vi "SA40289A.20211015 Data Analysis.vi"() -> ()   [LabVIEW 2020]
uses:
  <vilib>/Analysis/baseanly.llb/Mean (DBL).vi
  <userlib>/_OpenG.lib/file/file.llb/Build Path - Traditional__ogtk.vi
  <userlib>/LevyLab/XY Utilities/subVIs/Linear Fit (multiple).vi
  <userlib>/LevyLab/XY Utilities/subVIs/Get X and Y (multiple).vi
  <userlib>/LevyLab/LV to ITX/Data/Data.lvclass
  <userlib>/LevyLab/XY Utilities/xy_utilities.lvlib
  <vilib>/Analysis/NI_AALBase.lvlib
panel:
  out "Environment":enum16{"Air/Helium", "Vacuum"}(ring)
  out "Increasing Temp?":bool
  out "E_a":dbl[](array[numeric])
  in  "Tab Control":enum32{"2T data", "1D, 2D, and 4T Data"}(tab)
  out "G2T vs t":T1(graph)
  out "Temp vs t":T1(graph)
  out "G2T Slopes vs Temp":T1(graph)
  out "Arrhenius":T1(graph)
  out "G4T vs t 2D":T1(graph)
  out "G4T vs t 1D":T1(graph)
  out "Temp vs t 2":T1(graph)
  in  "One File?":bool
  in  "Arrhenius?":bool
  in  "2D Data?":bool=TRUE
  in  "Source Voltage":dbl=0.1
  in  "Init Temp":i32=275
  in  "Temp Step":i32=5
  in  "Final Temp":i32=300
  in  "Data File":path=path "G:/My Drive/ansom/Data (1)/PPMS 2/SA40289.20211015/00 - test/SA40289.20211015.275K.dat"
  in  "Trimming":i32=400
  in  "Update":bool
  in  "OK":bool
  out "error out":errorcluster
  in  "error in (no error)":errorcluster
  # "G2T"
  # "G4T 1D"
  # "G2T"
  # "G4T 2D"
  # "V1-"
  # "I-"
  # "V1+"
  # "V2-"
  # "I+"
  # "V2+"
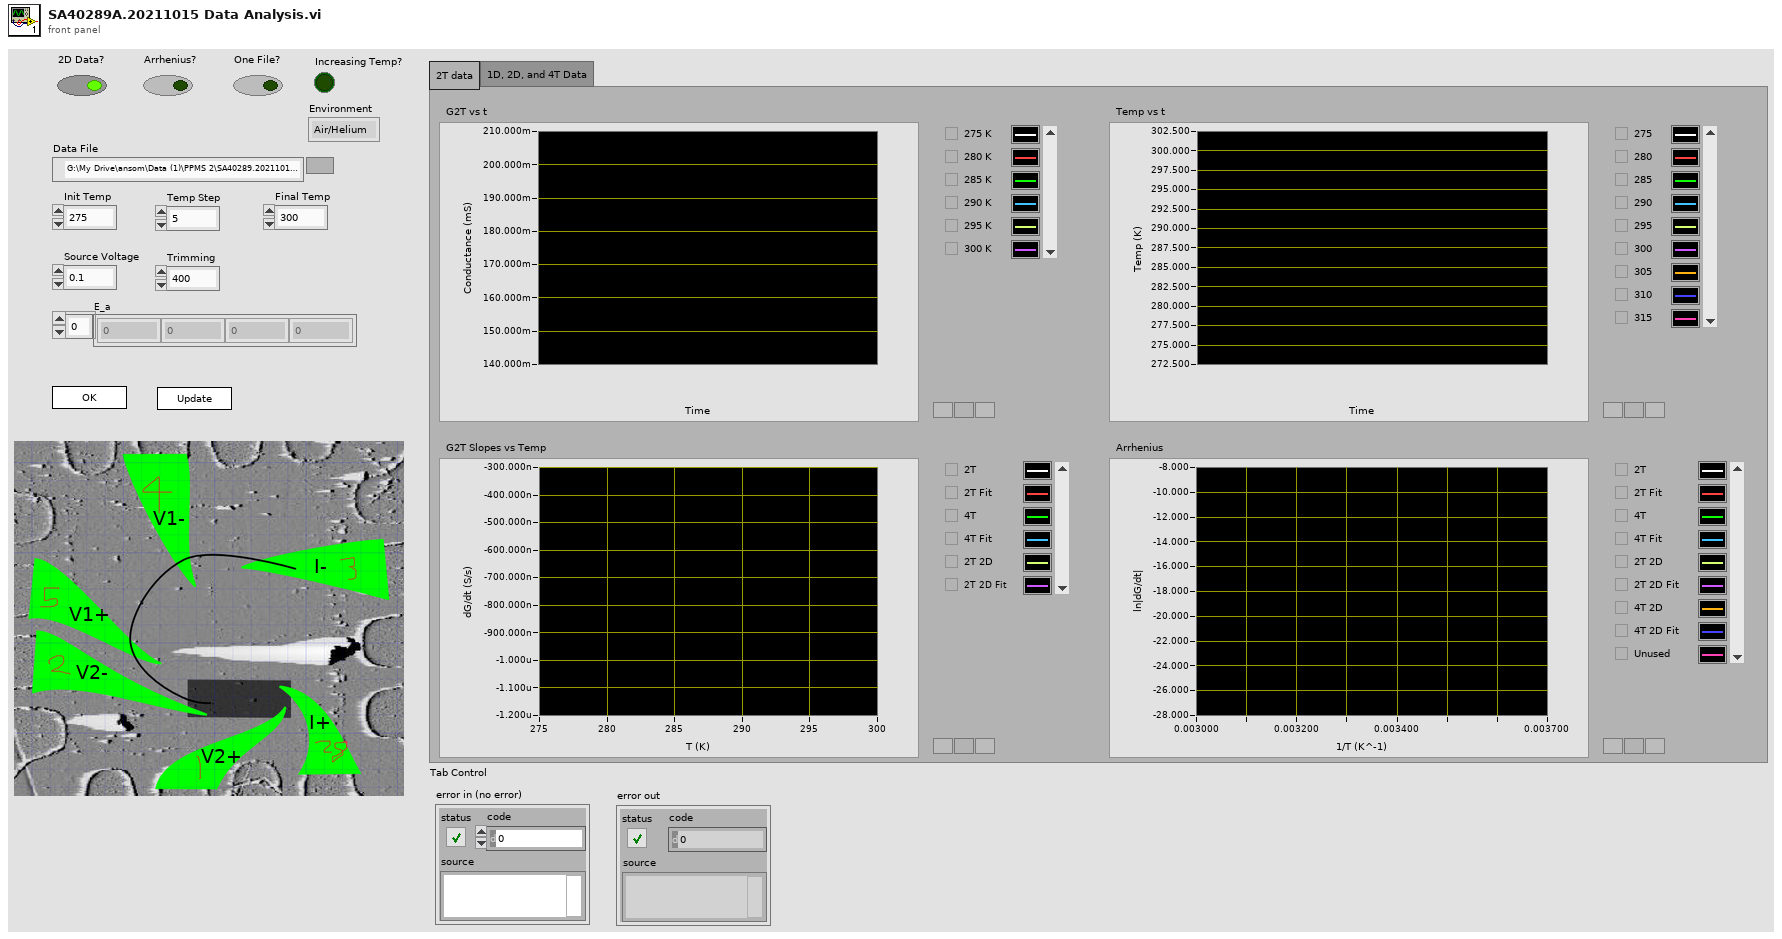
[diagram p1: front panel]
types:
  T1 = cluster{"Data":dbl[], "Best Exponential Fit":dbl[]}[]
  T2 = enum32{"Invalid", "Standard", "Closed", "Hidden", "Minimized", "Maximized"}
  T3 = enum32{"invalid app kind", "Development System", "Run Time System", "Student Edition", "Embedded LabVIEW", "Evaluation", "Custom"}
  T4 = cluster{"Core":cluster{"Current VI Reference":refnum<vi>, "Close Panel on Exit?":bool}, "G2T 1D":cluster{dbl[], dbl[]}[], "G4T 1D":cluster{dbl[], dbl[]}[], "G2T 2D":cluster{dbl[], dbl[]}[], "G4T 2D":cluster{dbl[], dbl[]}[], "Temp":cluster{dbl[], dbl[]}[], "G2T Slopes":cluster{dbl[], dbl[]}[], "Source Voltage":dbl, "Final Temp":i32, "Init Temp":i32, "Temp Step":i32, "Data File":path, "Trimming":i32}
  T5 = cluster{"Current VI Reference":refnum<vi>, "Close Panel on Exit?":bool}
  T6 = typedef "Data.lvclass/Dictionary--cluster.ctl" = cluster{"key":string, "value":variant}
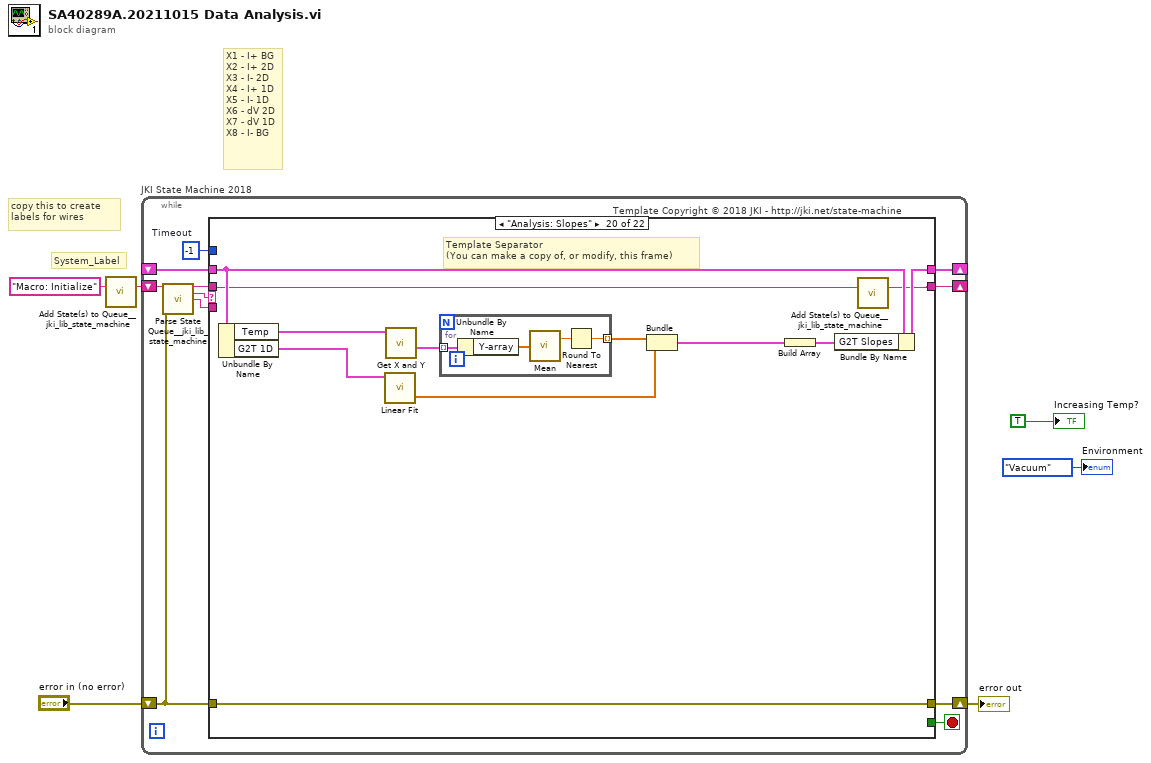
[diagram p0: block diagram]
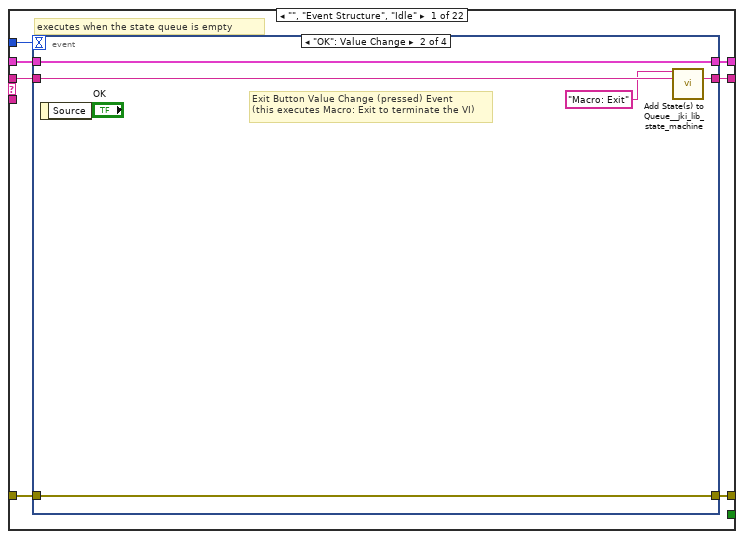
[diagram p2: hidden frame]
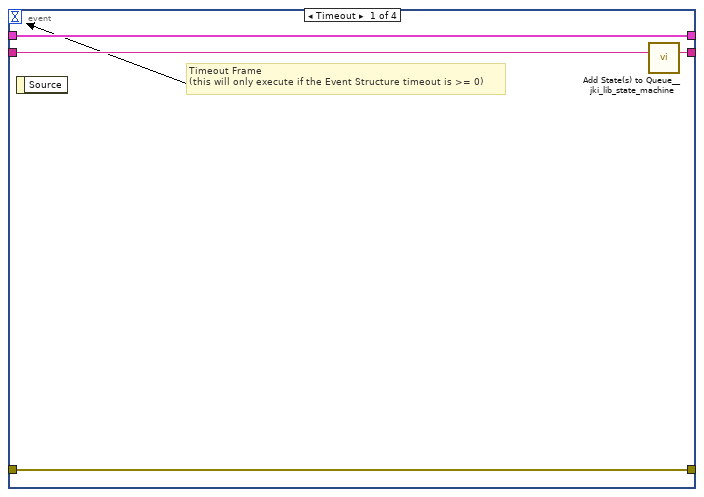
[diagram p3: hidden frame]
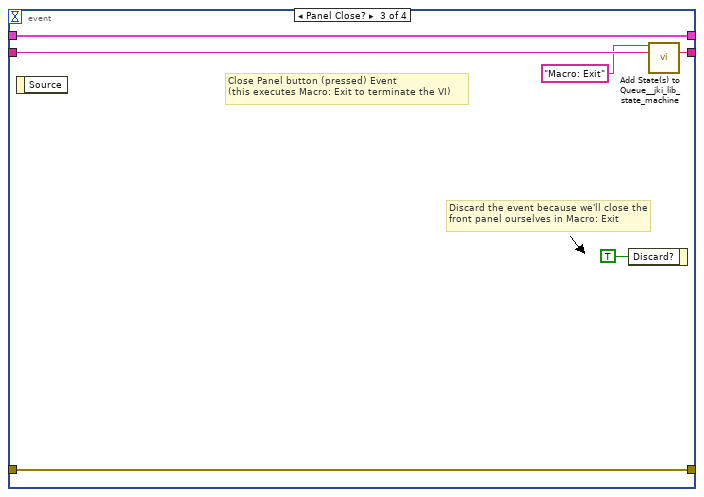
[diagram p4: hidden frame]
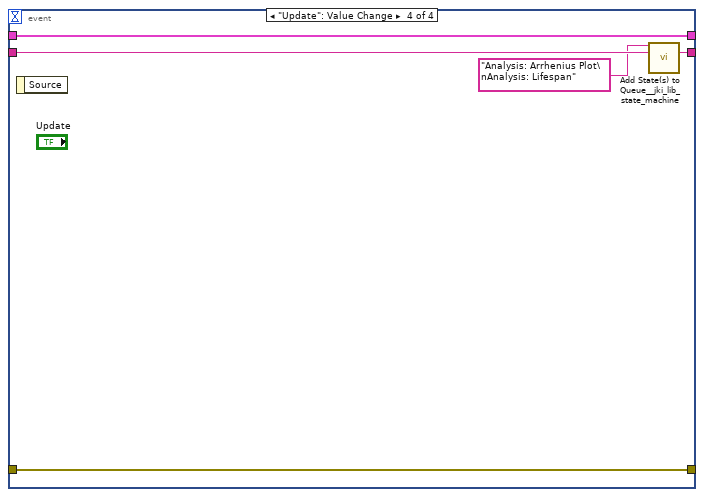
[diagram p5: hidden frame]
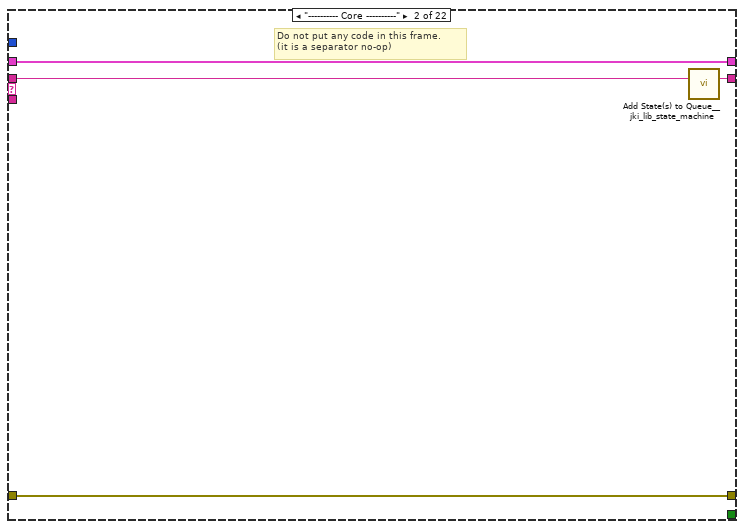
[diagram p6: hidden frame]
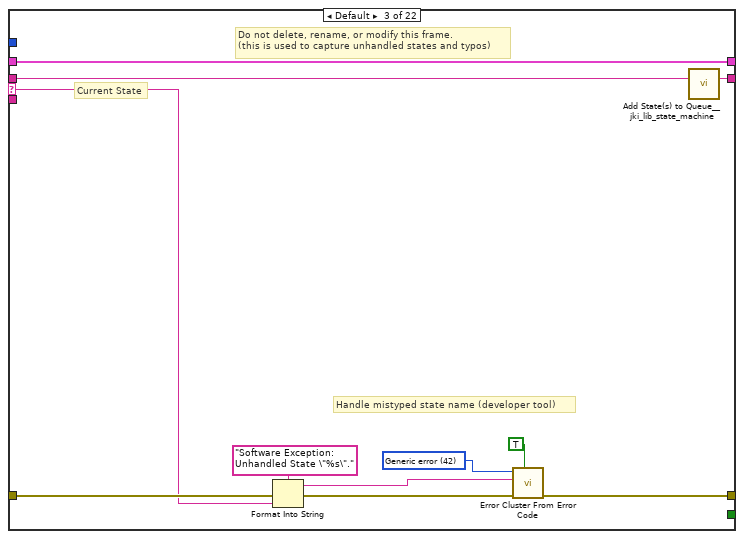
[diagram p7: hidden frame]
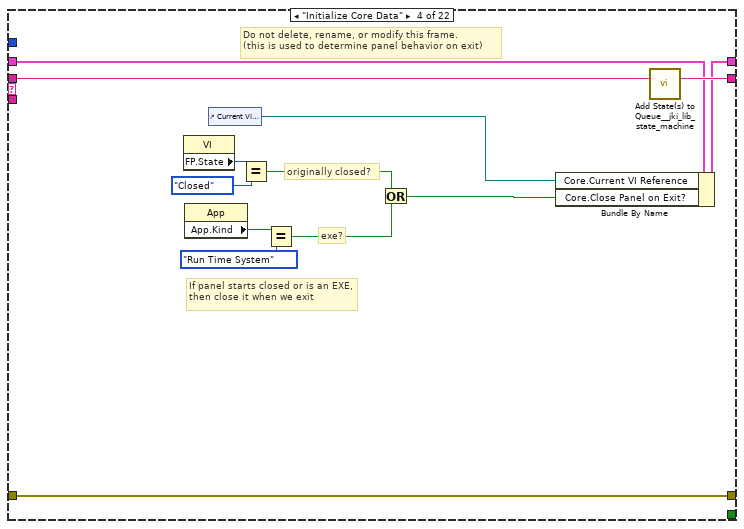
[diagram p8: hidden frame]
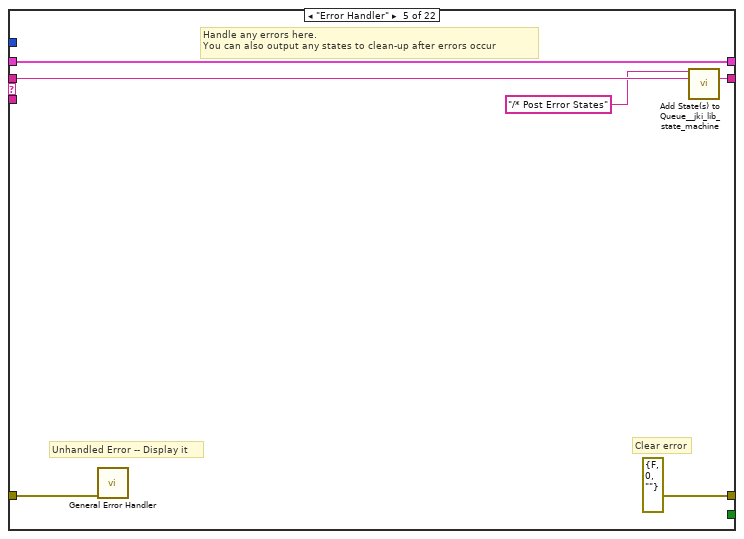
[diagram p9: hidden frame]
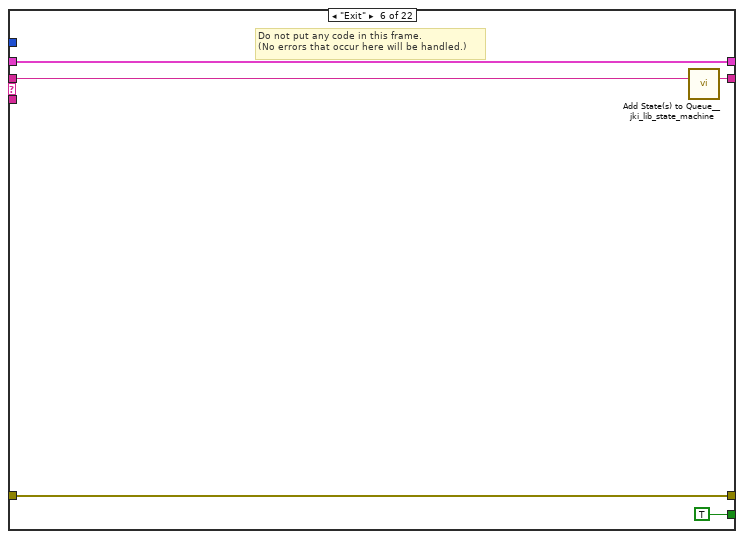
[diagram p10: hidden frame]
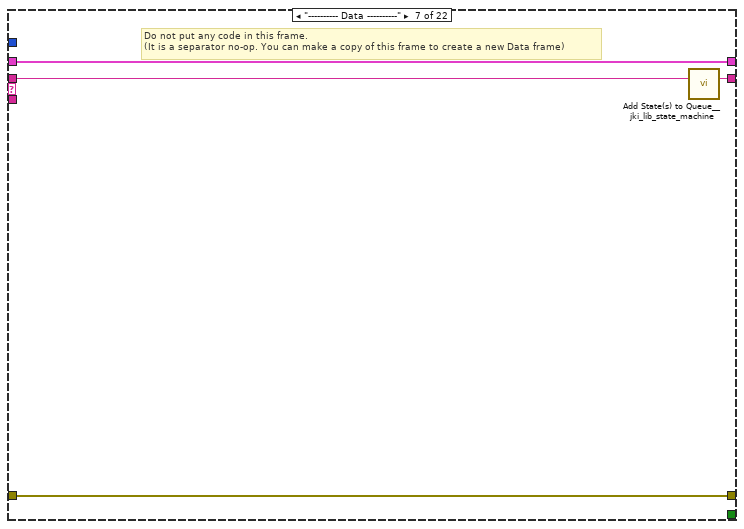
[diagram p11: hidden frame]
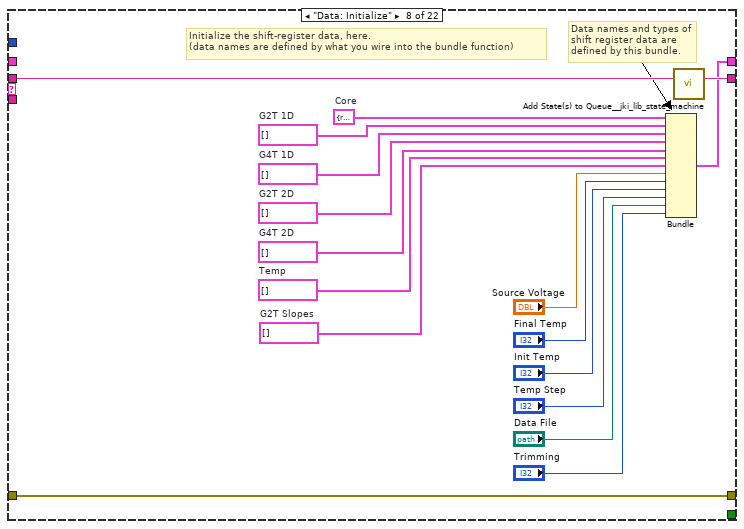
[diagram p12: hidden frame]
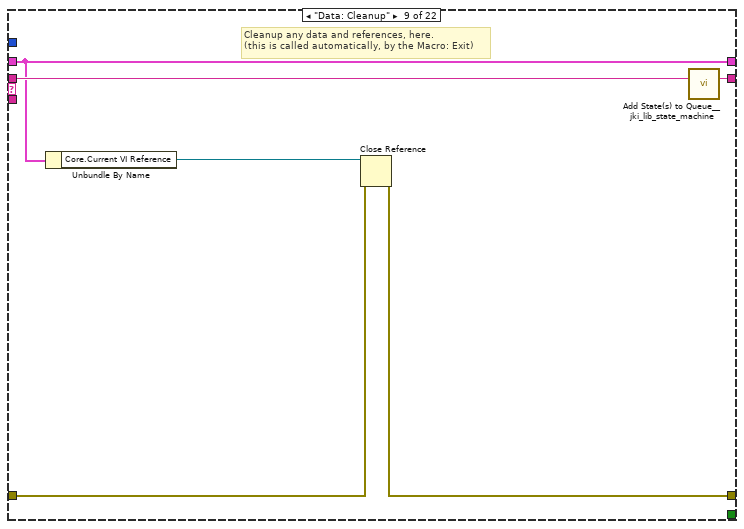
[diagram p13: hidden frame]
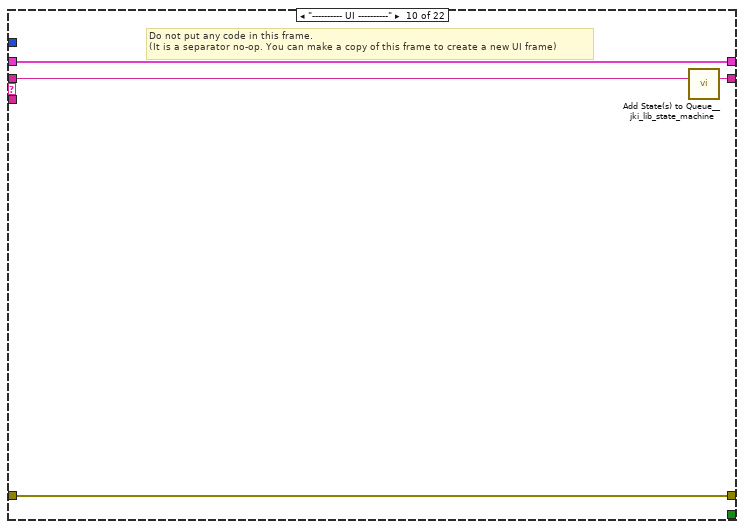
[diagram p14: hidden frame]
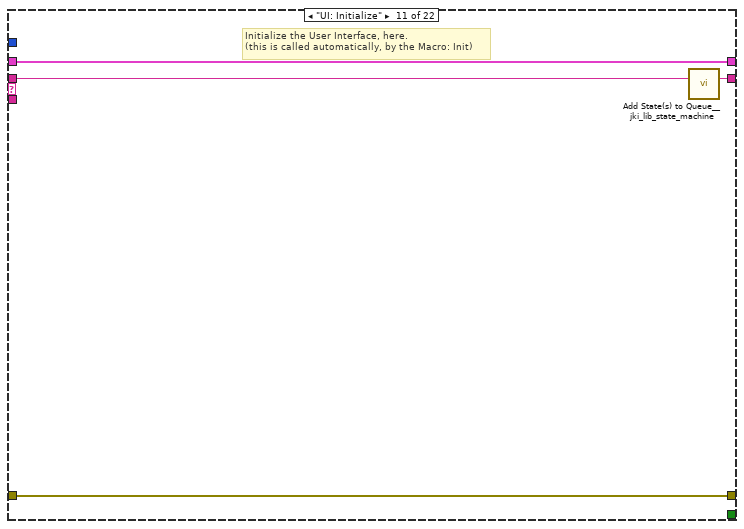
[diagram p15: hidden frame]
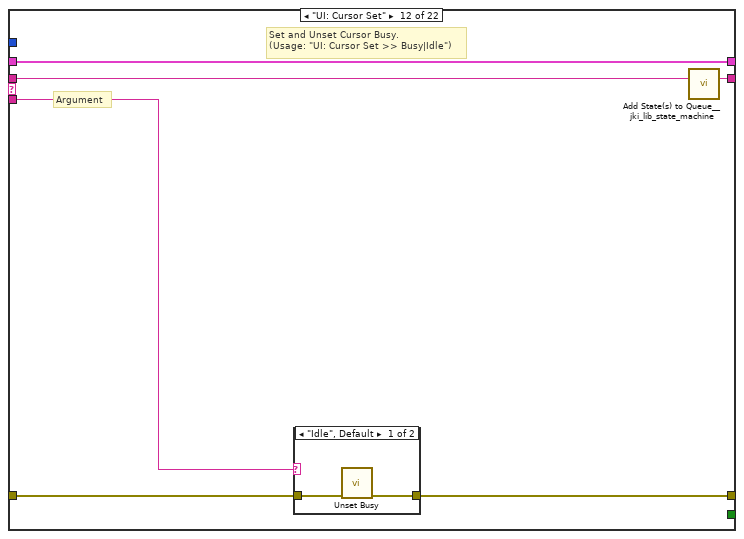
[diagram p16: hidden frame]
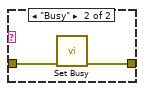
[diagram p17: hidden frame]
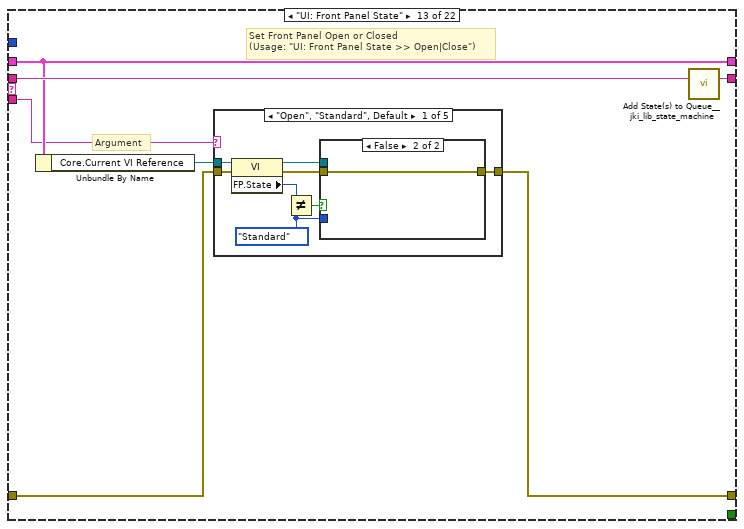
[diagram p18: hidden frame]
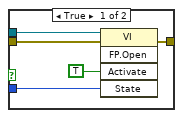
[diagram p19: hidden frame]
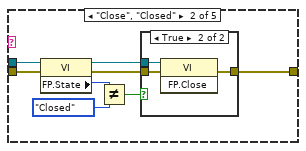
[diagram p20: hidden frame]
diagram:
  # "copy this to create labels for wires"
  # "System_Label"
  # "X1 - I+ BG\nX2 - I+ 2D\nX3 - I- 2D\nX4 - I+ 1D\nX5 - I- 1D\nX6 - dV 2D\nX7 - dV 1D\nX8 - I- BG"
  n1 = call <vilib>:"Add State(s) to Queue__jki_lib_state_machine.vi"("State(s) in (\"\")"="Macro: Initialize") -> ("States Out"=w6:string)  [unwired: 14 in]
  n2 = while "JKI State Machine 2018" {
    shift-right: [w10] -> _
    shift-left: _ -> [w9]
    shift-right: [w13] -> w3
    shift-left: "error in (no error)" -> [w7]
    shift-right: [w12] -> _
    shift-left: w6 -> [w14]
    stop <- w11 stop-if-true
    w8 = -1  # Timeout
    # "Template Copyright © 2018 JKI - http://jki.net/state-machine"
    n3 = call <vilib>:"Parse State Queue__jki_lib_state_machine.vi"("State Queue"=w14, "Error In (no error)"=w7) -> ("Remaining States"=w16:string, "Current State"=w17:string, "Arguments"=w15:string)  [unwired: 11 in]
    n4 = case shown="\"Analysis: Slopes\"" w17 {
      selector: w17 -> [_ _ w49 _ _ _ _ _ _ _ _ _ _ _ _ _ _ _ _ _ _ _]
      tunnel: w16 -> [w24 w48 w53 w72 w78 w83 w87 w104 w110 w114 w118 w124 w135 w204 w219 w229 w233 w250 w322 w371 w388 w446]
      tunnel: w15 -> [_ _ _ _ _ _ _ _ _ _ _ w119 w129 _ _ _ _ _ _ _ _ _]
      tunnel: w9 -> [w22 w45 w51 w65 w75 w81 w84 _ w105 w111 w116 w122 w131 w201 w216 w226 w230 w244 w308 w373 w385 w443]
      tunnel: [w21 w46 w55 w69 errorcluster {"status"=FALSE, "code"=0, "source"=""} ("error out") w80 w85 w101 w106 w112 w115 w120 w132 w202 w217 w227 w231 w246 w320 w375 w386 w444] -> w13
      tunnel: w7 -> [w20 w46 w54 w69 w74 w80 w85 w101 w107 w112 w115 w121 w133 w202 w217 w227 w231 w246 w320 w375 w386 w444]
      tunnel: [w23 w47 w52 w71 w77 w82 w86 w103 w109 w113 w117 w123 w134 w203 w218 w228 w232 w249 w321 w372 w387 w445] -> w12
      tunnel: [_ _ _ _ _ TRUE _ _ _ _ _ _ _ _ _ _ _ _ _ _ _ _] -> w11
      tunnel: [w19 w45 w51 w70 w75 w81 w84 w102 w105 w111 w116 w122 w131 w201 w216 w226 w230 w245 w309 w374 w385 w443] -> w10
      tunnel: w8 -> [w18 _ _ _ _ _ _ _ _ _ _ _ _ _ _ _ _ _ _ _ _ _]
      frame "", "Event Structure", "Idle" {
        # "executes when the state queue is empty"
        n5 = event shown="[1] \"OK\": Value Change" {
          selector: _ -> [_ _ _ _]
          dyn-events: _ -> [_ _ _ _]
          timeout: w18 -> [_ _ _ _]
          tunnel: w24 -> [w28 w33 w39 w43]
          tunnel: [w27 w32 w38 w42] -> w23
          tunnel: w22 -> [w25 w30 w36 w44]
          tunnel: [w26 w31 w37 w40] -> w21
          tunnel: w20 -> [w26 w31 w37 w40]
          tunnel: [w25 w30 w36 w44] -> w19
          event Timeout {
            # "Timeout Frame\n(this will only execute if the Event Structure timeout is >= 0)"
            n6 = event-data() -> ()  [unwired: 1 in, 1 out]
            n7 = call <vilib>:"Add State(s) to Queue__jki_lib_state_machine.vi"("State(s) in (\"\")"=w28) -> ("States Out"=w27:string)  [unwired: 14 in]
          }
          event "OK": Value Change {
            # "Exit Button Value Change (pressed) Event\n(this executes Macro: Exit to terminate the VI)"
            n8 = event-data() -> ()  [unwired: 1 in, 1 out]
            n9 = call <vilib>:"Add State(s) to Queue__jki_lib_state_machine.vi"("State(s) in Front (\"\")"="Macro: Exit", "State(s) in (\"\")"=w33) -> ("States Out"=w32:string)  [unwired: 13 in]
          }
          event Panel Close? {
            # "Discard the event because we'll close the front panel ourselves in Macro: Exit"
            # "Close Panel button (pressed) Event\n(this executes Macro: Exit to terminate the VI)"
            n10 = event-data() -> ()  [unwired: 1 in, 1 out]
            n11 = event-data("Discard?"=TRUE) -> ()  [unwired: 1 in, 1 out]
            n12 = call <vilib>:"Add State(s) to Queue__jki_lib_state_machine.vi"("State(s) in Front (\"\")"="Macro: Exit", "State(s) in (\"\")"=w39) -> ("States Out"=w38:string)  [unwired: 13 in]
          }
          event "Update": Value Change {
            n13 = event-data() -> ()  [unwired: 1 in, 1 out]
            n14 = call <vilib>:"Add State(s) to Queue__jki_lib_state_machine.vi"("State(s) in Front (\"\")"="Analysis: Arrhenius Plot\nAnalysis: Lifespan" ("State(s) in Front (\"\")"), "State(s) in (\"\")"=w43) -> ("States Out"=w42:string)  [unwired: 13 in]
          }
        }
      }
      frame "---------- Core ----------" {
        # "Do not put any code in this frame.\n(it is a separator no-op)"
        n15 = call <vilib>:"Add State(s) to Queue__jki_lib_state_machine.vi"("State(s) in (\"\")"=w48) -> ("States Out"=w47:string)  [unwired: 14 in]
      }
      frame Default {
        w58 = 42 items=["No error", "Argument error", "Memory is full", "Out of zone", "End of file", "File already open", "Generic file I/O error", "File not found", "File permission error", "Disk is full", "Duplicate path", "Too many files open", "System feature not enabled", "Resource file not found", "Cannot add resource", "Resource not found", "Image not found", "Image memory error", "Pen does not exist", "Config type invalid", "Config token not found", "Config parse error", "Config memory error", "Bad external code format", "Bad external code offset", "External code not present", "Null window", "Destroy window error", "Null menu", "Print aborted", "Bad print record", "Print driver error", "Windows error during printing", "Memory error during printing", "Print dialog error", "Generic print error", "Invalid device refnum", "Device not found", "Device parameter error", "Device unit error", "Cannot open device", "Device call aborted", "Generic error", "Cancelled by user", "Object ID too low", "Object ID too high", "Object not in heap", "Unknown heap", "Unknown object (invalid DefProc)", "Unknown object (DefProc not in table)", "Message out of range", "Invalid (null) method", "Unknown message", "Manager call not supported", "Bad address", "Network operation in progress", "Network operation timed out", "Connection is busy", "Network attribute not supported", "Network error", "Address in use", "System out of memory", "Connection aborted", "Connection refused", "Not connected", "Already connected", "Connection closed", "Initialization error (interapplication manager)", "Bad occurrence", "Wait on unbound occurrence handler", "Occurrence queue overflow", "Datalog type conflict", "Unused", "Unrecognized type (interapplication manager)", "Memory corrupt", "Failed to make temporary DLL", "Old CIN version", "Drag socket not found", "Failed to load drop-object", "Failed to register OLE object", "Failed to release OLE object", "Format specifier type mismatch", "Unknown format specifier", "Too few format specifiers", "Too many format specifiers", "Scan failed", "Newer CIN version", "Error converting to variant", "Runtime menu error", "Password tampered", "Variant attribute not found", "Incompatible variant data type", "Event data is not available", "Event Store is not present", "Occurrence is not found", "Event Queue is not created", "Event info is not available", "Refnum passed is NULL", "Error retrieving Class GUID", "Error retrieving CoClass GUID", "Error retrieving TypeLib GUID.", "Bad built application magic bytes.", "Specific driver is different from the specific driver associated with the Logical Name.", "There is no session opened to the class driver.", "Max Error", "MAX - Error with config objects", "MAX - Error loading configuration", "MAX - Group not supported"]
        # "Current State"
        # "Do not delete, rename, or modify this frame.\n(this is used to capture unhandled states and typos)"
        # "Handle mistyped state name (developer tool)"
        n16 = Format Into String(format string="Software Exception: Unhandled State \"%s\"." ("message"), error in=w54, w49) -> (resulting string=w57:string, error out=w56:errorcluster)  [unwired: 1 in]
        n17 = call <vilib>:"Error Cluster From Error Code.vi"("show call chain? (False)"=TRUE, "error in (no error)"=w56, "error message (\"\")"=w57, "error code (0)"=w58) -> ("error out"=w55:errorcluster)  [unwired: 5 in]
        n18 = call <vilib>:"Add State(s) to Queue__jki_lib_state_machine.vi"("State(s) in (\"\")"=w53) -> ("States Out"=w52:string)  [unwired: 14 in]
      }
      frame "Initialize Core Data" {
        # "Do not delete, rename, or modify this frame.\n(this is used to determine panel behavior on exit)"
        # "originally closed?"
        # "exe?"
        # "If panel starts closed or is an EXE, then close it when we exit"
        n19 = property class="VI"() -> ("FP.State"=w62:T2)  [unwired: 2 in, 2 out]
        n20 = property class="App"() -> ("App.Kind"=w68:T3)  [unwired: 2 in, 2 out]
        n21 = control-ref of="Current VI Reference"() -> (w63:refnum<vi>)
        n22 = Equal?(x=w62, y=T2."Closed" ("Front Panel Window:State")) -> (x = y?=w60:bool)
        n23 = Equal?(x=w68, y=T3."Run Time System" ("Application:Kind")) -> (x = y?=w66:bool)
        n24 = Or(x=w60, y=w66) -> (x .or. y?=w64:bool)
        n25 = Bundle By Name(cluster=w65, "Core.Current VI Reference"=w63, "Core.Close Panel on Exit?"=w64) -> (w70:T4)
        n26 = call <vilib>:"Add State(s) to Queue__jki_lib_state_machine.vi"("State(s) in (\"\")"=w72) -> ("States Out"=w71:string)  [unwired: 14 in]
      }
      frame "Error Handler" {
        # "Unhandled Error -- Display it"
        # "Handle any errors here.\nYou can also output any states to clean-up after errors occur"
        # "Clear error"
        n27 = call <vilib>:"General Error Handler.vi"("error in (no error)"=w74) -> ()  [unwired: 10 in, 5 out]
        n28 = call <vilib>:"Add State(s) to Queue__jki_lib_state_machine.vi"("State(s) in Front (\"\")"="/* Post Error States", "State(s) in (\"\")"=w78) -> ("States Out"=w77:string)  [unwired: 13 in]
      }
      frame "Exit" {
        # "Do not put any code in this frame.\n(No errors that occur here will be handled.)"
        n29 = call <vilib>:"Add State(s) to Queue__jki_lib_state_machine.vi"("State(s) in (\"\")"=w83) -> ("States Out"=w82:string)  [unwired: 14 in]
      }
      frame "---------- Data ----------" {
        # "Do not put any code in this frame.\n(It is a separator no-op. You can make a copy of this frame to create a new Data frame)"
        n30 = call <vilib>:"Add State(s) to Queue__jki_lib_state_machine.vi"("State(s) in (\"\")"=w87) -> ("States Out"=w86:string)  [unwired: 14 in]
      }
      frame "Data: Initialize" {
        w88 = cluster{dbl[], dbl[]}[] []  # G2T Slopes
        w89 = cluster{dbl[], dbl[]}[] []  # Temp
        w98 = cluster{dbl[], dbl[]}[] []  # G4T 2D
        w97 = cluster{dbl[], dbl[]}[] []  # G2T 2D
        w96 = cluster{dbl[], dbl[]}[] []  # G4T 1D
        w95 = cluster{dbl[], dbl[]}[] []  # G2T 1D
        w100 = T5 {"Current VI Reference"=refnum, "Close Panel on Exit?"=FALSE}  # Core
        # "Data names and types of shift register data are defined by this bundle."
        # "Initialize the shift-register data, here.\n(data names are defined by what you wire into the bundle function)"
        n31 = Bundle("Core"=w100, "G2T 1D"=w95, "G4T 1D"=w96, "G2T 2D"=w97, "G4T 2D"=w98, "Temp"=w89, "G2T Slopes"=w88, "Source Voltage"="Source Voltage", "Final Temp"="Final Temp", "Init Temp"="Init Temp", "Temp Step"="Temp Step", "Data File"="Data File", "Trimming"="Trimming") -> (w102:T4)  [unwired: 1 in]
        n32 = call <vilib>:"Add State(s) to Queue__jki_lib_state_machine.vi"("State(s) in (\"\")"=w104) -> ("States Out"=w103:string)  [unwired: 14 in]
      }
      frame "Data: Cleanup" {
        # "Cleanup any data and references, here.\n(this is called automatically, by the Macro: Exit)"
        n33 = Unbundle By Name(w105) -> ("Core.Current VI Reference"=w108:refnum<vi>)
        n34 = Close Reference(reference=w108, error in (no error)=w107) -> (error out=w106:errorcluster)
        n35 = call <vilib>:"Add State(s) to Queue__jki_lib_state_machine.vi"("State(s) in (\"\")"=w110) -> ("States Out"=w109:string)  [unwired: 14 in]
      }
      frame "---------- UI ----------" {
        # "Do not put any code in this frame.\n(It is a separator no-op. You can make a copy of this frame to create a new UI frame)"
        n36 = call <vilib>:"Add State(s) to Queue__jki_lib_state_machine.vi"("State(s) in (\"\")"=w114) -> ("States Out"=w113:string)  [unwired: 14 in]
      }
      frame "UI: Initialize" {
        # "Initialize the User Interface, here.\n(this is called automatically, by the Macro: Init)"
        n37 = call <vilib>:"Add State(s) to Queue__jki_lib_state_machine.vi"("State(s) in (\"\")"=w118) -> ("States Out"=w117:string)  [unwired: 14 in]
      }
      frame "UI: Cursor Set" {
        # "Argument"
        # "Set and Unset Cursor Busy.\n(Usage: \"UI: Cursor Set >> Busy|Idle\")"
        n38 = case shown="\"Idle\", Default" w119 {
          tunnel: w121 -> [w126 w128]
          tunnel: [w125 w127] -> w120
          frame "Idle", Default {
            n39 = call <vilib>:"Unset Busy.vi"("error in (no error)"=w126) -> ("error out"=w125:errorcluster)  [unwired: 10 in]
          }
          frame "Busy" {
            n40 = call <vilib>:"Set Busy.vi"("error in (no error)"=w128) -> ("error out"=w127:errorcluster)  [unwired: 9 in, 1 out]
          }
        }
        n41 = call <vilib>:"Add State(s) to Queue__jki_lib_state_machine.vi"("State(s) in (\"\")"=w124) -> ("States Out"=w123:string)  [unwired: 14 in]
      }
      frame "UI: Front Panel State" {
        # "Argument"
        # "Set Front Panel Open or Closed\n(Usage: \"UI: Front Panel State >> Open|Close\")"
        n42 = Unbundle By Name(w131) -> ("Core.Current VI Reference"=w130:refnum<vi>)
        n43 = case shown="\"Open\", \"Standard\", Default" w129 {
          tunnel: w133 -> [w141 w156 w167 w180 w193]
          tunnel: [w143 w157 w169 w182 w195] -> w132
          tunnel: w130 -> [w142 w154 w168 w181 w194]
          frame "Open", "Standard", Default {
            w136 = T2."Standard" ("State")
            n44 = property class="VI"(reference=w142, error in=w141) -> (reference out=w139:refnum<vi>, error out=w140:errorcluster, "FP.State"=w138:T2)
            n45 = Not Equal?(x=w138, y=w136) -> (x != y?=w137:bool)
            n46 = case shown="False" w137 {
              tunnel: [w147 w149] -> w143
              tunnel: w140 -> [w146 w149]
              tunnel: w139 -> [w145 _]
              tunnel: w136 -> [w144 _]
              frame True {
                n47 = invoke class="VI" method="FP.Open"(reference=w145, error in=w146, "Activate"=TRUE, "State"=w144) -> (error out=w147:errorcluster)  [unwired: 1 in, 4 out]
              }
              frame False {
              }
            }
          }
          frame "Close", "Closed" {
            n48 = property class="VI"(reference=w154, error in=w156) -> (reference out=w153:refnum<vi>, error out=w155:errorcluster, "FP.State"=w151:T2)
            n49 = Not Equal?(x=w151, y=T2."Closed" ("Front Panel Window:State")) -> (x != y?=w150:bool)
            n50 = case shown="True" w150 {
              tunnel: [w158 w161] -> w157
              tunnel: w155 -> [w158 w160]
              tunnel: w153 -> [_ w159]
              frame False {
              }
              frame True {
                n51 = invoke class="VI" method="FP.Close"(reference=w159, error in=w160) -> (error out=w161:errorcluster)  [unwired: 1 in, 2 out]
              }
            }
          }
          frame "Hidden", "Hide" {
            w162 = T2."Hidden" ("State")
            n52 = property class="VI"(reference=w168, error in=w167) -> (reference out=w165:refnum<vi>, error out=w166:errorcluster, "FP.State"=w164:T2)
            n53 = Not Equal?(x=w164, y=w162) -> (x != y?=w163:bool)
            n54 = case shown="True" w163 {
              tunnel: [w173 w174] -> w169
              tunnel: w166 -> [w172 w174]
              tunnel: w165 -> [w171 _]
              tunnel: w162 -> [w170 _]
              frame True {
                n55 = invoke class="VI" method="FP.Open"(reference=w171, error in=w172, "State"=w170) -> (error out=w173:errorcluster)  [unwired: 2 in, 4 out]
              }
              frame False {
              }
            }
          }
          frame "Minimize", "Minimized" {
            w175 = T2."Minimized" ("State")
            n56 = property class="VI"(reference=w181, error in=w180) -> (reference out=w178:refnum<vi>, error out=w179:errorcluster, "FP.State"=w177:T2)
            n57 = Not Equal?(x=w177, y=w175) -> (x != y?=w176:bool)
            n58 = case shown="True" w176 {
              tunnel: [w186 w187] -> w182
              tunnel: w179 -> [w185 w187]
              tunnel: w178 -> [w184 _]
              tunnel: w175 -> [w183 _]
              frame True {
                n59 = invoke class="VI" method="FP.Open"(reference=w184, error in=w185, "State"=w183) -> (error out=w186:errorcluster)  [unwired: 2 in, 4 out]
              }
              frame False {
              }
            }
          }
          frame "Maximize", "Maximized" {
            w188 = T2."Maximized" ("State")
            n60 = property class="VI"(reference=w194, error in=w193) -> (reference out=w191:refnum<vi>, error out=w192:errorcluster, "FP.State"=w190:T2)
            n61 = Not Equal?(x=w190, y=w188) -> (x != y?=w189:bool)
            n62 = case shown="True" w189 {
              tunnel: [w199 w200] -> w195
              tunnel: w192 -> [w198 w200]
              tunnel: w191 -> [w197 _]
              tunnel: w188 -> [w196 _]
              frame True {
                n63 = invoke class="VI" method="FP.Open"(reference=w197, error in=w198, "State"=w196) -> (error out=w199:errorcluster)  [unwired: 2 in, 4 out]
              }
              frame False {
              }
            }
          }
        }
        n64 = call <vilib>:"Add State(s) to Queue__jki_lib_state_machine.vi"("State(s) in (\"\")"=w135) -> ("States Out"=w134:string)  [unwired: 14 in]
      }
      frame "---------- Macro ----------" {
        # "Do not put any code in this frame.\n(It is a separator no-op. You can make a copy of this frame to create a new Macro frame)"
        n65 = call <vilib>:"Add State(s) to Queue__jki_lib_state_machine.vi"("State(s) in (\"\")"=w204) -> ("States Out"=w203:string)  [unwired: 14 in]
      }
      frame "Macro: Initialize" {
        w213 = ""
        # "Initialization Macro\n(This is called once, when the VI starts)"
        n66 = Select(t="Analysis: 2D Data", s="2D Data?", f=w213) -> (s? t:f=w206:string)
        n67 = Select(t="Analysis: Arrhenius Plot", s="Arrhenius?", f=w213) -> (s? t:f=w205:string)
        n68 = call <vilib>:"Add State(s) to Queue__jki_lib_state_machine.vi"("State(s) in Front (\"\")"=w206, "State(s) in (\"\")"=w205, "State(s) at Back (\"\")"="Analysis: Plot G vs t") -> ("States Out"=w209:string)  [unwired: 12 in]
        n69 = call <vilib>:"Add State(s) to Queue__jki_lib_state_machine.vi"("State(s) in Front (\"\")"="Data: Initialize\nInitialize Core Data\nUI: Initialize\nUI: Front Panel State >> Open\nAnalysis: Load 1D\nAnalysis: Slopes\n", "State(s) at Back (\"\")"=w209) -> ("States Out"=w207:string)  [unwired: 13 in]
        n70 = call <vilib>:"Add State(s) to Queue__jki_lib_state_machine.vi"("State(s) in Front (\"\")"=w207, "State(s) in (\"\")"=w219) -> ("States Out"=w218:string)  [unwired: 13 in]
      }
      frame "Macro: Exit" {
        # "Exit Macro\n(This is called once, when the VI exits)"
        n71 = Unbundle By Name(w226) -> ("Core.Close Panel on Exit?"=w225:bool)
        n72 = Select(t="UI: Front Panel State >> Close", s=w225, f="") -> (s? t:f=w222:string)
        n73 = call <vilib>:"Add State(s) to Queue__jki_lib_state_machine.vi"("State(s) in (\"\")"=w222, "State(s) at Back (\"\")"="Data: Cleanup\nExit") -> ("States Out"=w220:string)  [unwired: 13 in]
        n74 = call <vilib>:"Add State(s) to Queue__jki_lib_state_machine.vi"("State(s) in Front (\"\")"=w220, "State(s) in (\"\")"=w229) -> ("States Out"=w228:string)  [unwired: 13 in]
      }
      frame "---------- Analysis ----------" {
        # "Template Separator\n(You can make a copy of, or modify, this frame)"
        n75 = call <vilib>:"Add State(s) to Queue__jki_lib_state_machine.vi"("State(s) in (\"\")"=w233) -> ("States Out"=w232:string)  [unwired: 14 in]
      }
      frame "Analysis: Load 1D" {
        n76 = Unbundle By Name(w244) -> ("Source Voltage"=w243:dbl, "Final Temp"=w242:i32, "Init Temp"=w239:i32, "Temp Step"=w238:i32, "Data File"=w240:path, "Trimming"=w237:i32)
        n77 = Subtract(x=w242, y=w239) -> (x-y=w247:i32)
        n78 = Divide(x=w247, y=w238) -> (x/y=w248:dbl)
        n79 = Increment(x=w248) -> (x+1=w241:dbl)
        n80 = case shown="True" "One File?" {
          tunnel: w243 -> [w258 w296]
          tunnel: w241 -> [w256 _]
          tunnel: w240 -> [w255 w295]
          tunnel: w239 -> [w254 _]
          tunnel: w238 -> [w253 _]
          tunnel: w237 -> [w252 w289]
          tunnel: [w251 w293] -> w236
          tunnel: [w257 w291] -> w234
          frame False {
            n81 = for {
              N: w256 -> [_]
              tunnel: w258 -> [w265]
              tunnel: [w276] -> w257 mode=indexing
              tunnel: w255 -> [w275]
              tunnel: w254 -> [w274]
              tunnel: w253 -> [w273]
              tunnel: w252 -> [w259]
              tunnel: [w271] -> w251 mode=indexing
              i -> [w279]
              n82 = Strip Path(path=w275) -> (stripped path=w284:path, name=w283:string)
              n83 = Multiply(x=w273, y=w279) -> (x*y=w280:i32)
              n84 = Add(x=w274, y=w280) -> (x+y=w285:i32)
              n85 = String Subset(string=w283, length (rest)=17) -> (substring=w281:string)  [unwired: 1 in]
              n86 = Format Into String(w285) -> (resulting string=w287:string)  [unwired: 3 in, 1 out]
              n87 = Concatenate Strings(w281, w287, "K.dat" ("string")) -> (w286:string)
              n88 = call-poly <userlib>:"Build Path__ogtk.vi"("name or relative path"=w286, "base path"=w284) -> ("appended path"=w288:path)
              n89 = call <userlib>:"Data Read.vi"("path"=w288) -> ("Data (Dictionary)"=w262:T6[])  [unwired: 7 in, 3 out]
              n90 = call "Read Dictionary.vi"("Numeric"=0, "Dictionary In"=w262) -> ("data"=w268:dbl[])
              n91 = call "Read Dictionary.vi"("Numeric"=5 ("index"), "Dictionary In"=w262) -> ("data"=w266:dbl[])
              n92 = call "Read Dictionary.vi"("Numeric"=1, "Dictionary In"=w262) -> ("data"=w261:dbl[])
              n93 = Array Subset(array=w261, index=w259) -> (w260:dbl[])  [unwired: 1 in]
              n94 = Array Subset(array=w268, index=w259) -> (w272:dbl[])  [unwired: 1 in]
              n95 = Array Subset(array=w266, index=w259) -> (w264:dbl[])  [unwired: 1 in]
              n96 = Divide(x=w264, y=w265) -> (x/y=w278:dbl[])
              n97 = Absolute Value(x=w278) -> (abs(x)=w263:dbl[])
              n98 = Bundle(w272, w263) -> (w276:cluster{dbl[], dbl[]})  [unwired: 1 in]
              n99 = Bundle(w272, w260) -> (w271:cluster{dbl[], dbl[]})  [unwired: 1 in]
            }
          }
          frame True {
            n100 = call <userlib>:"Data Read.vi"("path"=w295) -> ("Data (Dictionary)"=w297:T6[])  [unwired: 7 in, 3 out]
            n101 = call "Read Dictionary.vi"("Numeric"=0, "Dictionary In"=w297) -> ("data"=w302:dbl[])
            n102 = call "Read Dictionary.vi"("Numeric"=5 ("index"), "Dictionary In"=w297) -> ("data"=w290:dbl[])
            n103 = call "Read Dictionary.vi"("Numeric"=1, "Dictionary In"=w297) -> ("data"=w301:dbl[])
            n104 = Array Subset(array=w302, index=w289) -> (w306:dbl[])  [unwired: 1 in]
            n105 = Array Subset(array=w290, index=w289) -> (w299:dbl[])  [unwired: 1 in]
            n106 = Array Subset(array=w301, index=w289) -> (w305:dbl[])  [unwired: 1 in]
            n107 = Divide(x=w299, y=w296) -> (x/y=w307:dbl[])
            n108 = Absolute Value(x=w307) -> (abs(x)=w298:dbl[])
            n109 = Bundle(w306, w298) -> (w292:cluster{dbl[], dbl[]})  [unwired: 1 in]
            n110 = Bundle(w306, w305) -> (w294:cluster{dbl[], dbl[]})  [unwired: 1 in]
            n111 = Build Array(w292) -> (w291:cluster{dbl[], dbl[]}[])
            n112 = Build Array(w294) -> (w293:cluster{dbl[], dbl[]}[])
          }
        }
        n113 = call <vilib>:"Add State(s) to Queue__jki_lib_state_machine.vi"("State(s) in (\"\")"=w250) -> ("States Out"=w249:string)  [unwired: 14 in]
        n114 = Bundle By Name(cluster=w244, "G2T 1D"=w234, "Temp"=w236) -> (w245:T4)
      }
      frame "Analysis: 2D Data" {
        n115 = Unbundle By Name(w308) -> ("Final Temp"=w315:i32, "Init Temp"=w312:i32, "Temp Step"=w311:i32, "Data File"=w313:path, "Trimming"=w310:i32)
        n116 = Subtract(x=w315, y=w312) -> (x-y=w318:i32)
        n117 = Divide(x=w318, y=w311) -> (x/y=w319:dbl)
        n118 = Increment(x=w319) -> (x+1=w314:dbl)
        n119 = for {
          N: w314 -> [_]
          tunnel: [w351] -> w317 mode=indexing
          tunnel: [w350] -> w316 mode=indexing
          tunnel: w313 -> [w349]
          tunnel: w312 -> [w348]
          tunnel: w311 -> [w347]
          tunnel: w310 -> [w331]
          i -> [w354]
          n120 = Strip Path(path=w349) -> (stripped path=w359:path, name=w358:string)
          n121 = Multiply(x=w347, y=w354) -> (x*y=w355:i32)
          n122 = Add(x=w348, y=w355) -> (x+y=w360:i32)
          n123 = String Subset(string=w358, length (rest)=17) -> (substring=w356:string)  [unwired: 1 in]
          n124 = Format Into String(w360) -> (resulting string=w362:string)  [unwired: 3 in, 1 out]
          n125 = Concatenate Strings(w356, w362, "K.dat" ("string")) -> (w361:string)
          n126 = call-poly <userlib>:"Build Path__ogtk.vi"("name or relative path"=w361, "base path"=w359) -> ("appended path"=w363:path)
          n127 = call <userlib>:"Data Read.vi"("path"=w363) -> ("Data (Dictionary)"=w325:T6[])  [unwired: 7 in, 3 out]
          n128 = call "Read Dictionary.vi"("Numeric"=0, "Dictionary In"=w325) -> ("data"=w345:dbl[])
          n129 = call "Read Dictionary.vi"("Numeric"=5 ("index"), "Dictionary In"=w325) -> ("data"=w337:dbl[])
          n130 = call "Read Dictionary.vi"("Numeric"=6 ("index"), "Dictionary In"=w325) -> ("data"=w330:dbl[])
          n131 = call "Read Dictionary.vi"("Numeric"=7, "Dictionary In"=w325) -> ("data"=w332:dbl[])
          n132 = call "Read Dictionary.vi"("Numeric"=4 ("index"), "Dictionary In"=w325) -> ("data"=w343:dbl[])
          n133 = call "Read Dictionary.vi"("Numeric"=3, "Dictionary In"=w325) -> ("data"=w344:dbl[])
          n134 = Array Subset(array=w345, index=w331) -> (w346:dbl[])  [unwired: 1 in]
          n135 = Array Subset(array=w337, index=w331) -> (w324:dbl[])  [unwired: 1 in]
          n136 = Array Subset(array=w330, index=w331) -> (w329:dbl[])  [unwired: 1 in]
          n137 = Array Subset(array=w332, index=w331) -> (w328:dbl[])  [unwired: 1 in]
          n138 = Array Subset(array=w343, index=w331) -> (w336:dbl[])  [unwired: 1 in]
          n139 = Array Subset(array=w344, index=w331) -> (w335:dbl[])  [unwired: 1 in]
          n140 = Subtract(x=w336, y=w335) -> (x-y=w323:dbl[])
          n141 = Subtract(x=w329, y=w328) -> (x-y=w327:dbl[])
          n142 = Divide(x=w324, y=w327) -> (x/y=w326:dbl[])
          n143 = Divide(x=w323, y=w324) -> (x/y=w353:dbl[])
          n144 = Bundle(w346, w326) -> (w351:cluster{dbl[], dbl[]})  [unwired: 1 in]
          n145 = Absolute Value(x=w353) -> (abs(x)=w339:dbl[])
          n146 = Bundle(w346, w339) -> (w350:cluster{dbl[], dbl[]})  [unwired: 1 in]
        }
        n147 = call <vilib>:"Add State(s) to Queue__jki_lib_state_machine.vi"("State(s) in (\"\")"=w322) -> ("States Out"=w321:string)  [unwired: 14 in]
        n148 = Bundle By Name(cluster=w308, "G4T 1D"=w317, "G4T 2D"=w316) -> (w309:T4)
      }
      frame "Analysis: Slopes" {
        # "Template Separator\n(You can make a copy of, or modify, this frame)"
        n149 = Unbundle By Name(w373) -> ("Temp"=w366:cluster{dbl[], dbl[]}[], "G2T 1D"=w369:cluster{dbl[], dbl[]}[])
        n150 = call-poly <userlib>:"Linear Fit.vi"("XY-data"=w369) -> ("slopes"=w368:dbl[])  [unwired: 4 in, 6 out]
        n151 = call-poly <userlib>:"Get X and Y.vi"("XY-data"=w366) -> ("Y-Arrays"=w365:cluster{"Y-array":dbl[]}[])  [unwired: 7 in, 3 out]
        n152 = for {
          tunnel: w365 -> [w379] mode=indexing
          tunnel: [w376] -> w364 mode=indexing
          n153 = Unbundle By Name(w379) -> ("Y-array"=w378:dbl[])
          n154 = call-poly <vilib>:"Mean.vi"("X"=w378) -> ("mean"=w377:dbl)  [unwired: 1 out]
          n155 = Round To Nearest(number=w377) -> (nearest integer value=w376:dbl)
        }
        n156 = Bundle(w364, "slopes"=w368) -> (w367:cluster{dbl[], "slopes":dbl[]})  [unwired: 1 in]
        n157 = Build Array(w367) -> (w370:cluster{dbl[], "slopes":dbl[]}[])
        n158 = Bundle By Name(cluster=w373, "G2T Slopes"=w370) -> (w374:T4)
        n159 = call <vilib>:"Add State(s) to Queue__jki_lib_state_machine.vi"("State(s) in (\"\")"=w371) -> ("States Out"=w372:string)  [unwired: 14 in]
      }
      frame "Analysis: Plot G vs t" {
        n160 = Unbundle By Name(w385) -> ("G2T 1D"=→"G2T vs t":cluster{dbl[], dbl[]}[], "G4T 1D"=→"G4T vs t 1D":cluster{dbl[], dbl[]}[], "Temp"=→"Temp vs t" →"Temp vs t 2":cluster{dbl[], dbl[]}[], "G2T Slopes"=→"G2T Slopes vs Temp":cluster{dbl[], dbl[]}[], "G4T 2D"=→"G4T vs t 2D":cluster{dbl[], dbl[]}[])
        n161 = call <vilib>:"Add State(s) to Queue__jki_lib_state_machine.vi"("State(s) in (\"\")"=w388) -> ("States Out"=w387:string)  [unwired: 14 in]
      }
      frame "Analysis: Arrhenius Plot" {
        n162 = Unbundle By Name(w443) -> ("G2T 1D"=w411:cluster{dbl[], dbl[]}[], "G4T 1D"=w410:cluster{dbl[], dbl[]}[], "G2T 2D"=w417:cluster{dbl[], dbl[]}[], "G4T 2D"=w419:cluster{dbl[], dbl[]}[], "Final Temp"=w440:i32, "Init Temp"=w438:i32, "Temp Step"=w437:i32)  [unwired: 1 out]
        n163 = Subtract(x=w440, y=w438) -> (x-y=w441:i32)
        n164 = Divide(x=w441, y=w437) -> (x/y=w442:dbl)
        n165 = Increment(x=w442) -> (x+1=w439:dbl)
        n166 = for {
          N: w439 -> [_]
          tunnel: w438 -> [w449]
          tunnel: w437 -> [w450]
          tunnel: [w447] -> w427 mode=indexing
          i -> [w451]
          n167 = Multiply(x=w450, y=w451) -> (x*y=w452:i32)
          n168 = Add(x=w449, y=w452) -> (x+y=w448:i32)
          n169 = Reciprocal(x=w448) -> (1/x=w447:dbl)
        }
        n170 = call-poly <userlib>:"Linear Fit.vi"("XY-data"=w411) -> ("XY-data out"=w406:cluster{"X-array":dbl[], "Y-array":dbl[]}[], "slopes"=w408:dbl[])  [unwired: 4 in, 5 out]
        n171 = call-poly <userlib>:"Linear Fit.vi"("XY-data"=w410) -> ("XY-data out"=w395:cluster{"X-array":dbl[], "Y-array":dbl[]}[], "slopes"=w409:dbl[])  [unwired: 4 in, 5 out]
        n172 = call-poly <userlib>:"Linear Fit.vi"("XY-data"=w417) -> ("XY-data out"=w396:cluster{"X-array":dbl[], "Y-array":dbl[]}[], "slopes"=w416:dbl[])  [unwired: 4 in, 5 out]
        n173 = call-poly <userlib>:"Linear Fit.vi"("XY-data"=w419) -> ("XY-data out"=w397:cluster{"X-array":dbl[], "Y-array":dbl[]}[], "slopes"=w418:dbl[])  [unwired: 4 in, 5 out]
        n174 = Absolute Value(x=w408) -> (abs(x)=w405:dbl[])
        n175 = Absolute Value(x=w409) -> (abs(x)=w399:dbl[])
        n176 = Absolute Value(x=w416) -> (abs(x)=w400:dbl[])
        n177 = Absolute Value(x=w418) -> (abs(x)=w398:dbl[])
        n178 = call <userlib>:"Average.vi"("XY-data"=w406) -> ("Averaged XY-data out"=w407:cluster{"X-array":dbl[], "Y-array":dbl[]})  [unwired: 8 in, 2 out]
        n179 = call <userlib>:"Average.vi"("XY-data"=w395) -> ("Averaged XY-data out"=w394:cluster{"X-array":dbl[], "Y-array":dbl[]})  [unwired: 8 in, 2 out]
        n180 = call <userlib>:"Average.vi"("XY-data"=w396) -> ("Averaged XY-data out"=w392:cluster{"X-array":dbl[], "Y-array":dbl[]})  [unwired: 8 in, 2 out]
        n181 = call <userlib>:"Average.vi"("XY-data"=w397) -> ("Averaged XY-data out"=w393:cluster{"X-array":dbl[], "Y-array":dbl[]})  [unwired: 8 in, 2 out]
        n182 = Unbundle(w407) -> ("Y-array"=w404:dbl[])  [unwired: 1 out]
        n183 = Unbundle(w394) -> ("Y-array"=w389:dbl[])  [unwired: 1 out]
        n184 = Unbundle(w393) -> ("Y-array"=w391:dbl[])  [unwired: 1 out]
        n185 = Unbundle(w392) -> ("Y-array"=w390:dbl[])  [unwired: 1 out]
        n186 = Divide(x=w405, y=w404) -> ()  [unwired: 1 out]
        n187 = Divide(x=w399, y=w389) -> (x/y=w401:dbl[])
        n188 = Divide(x=w400, y=w390) -> (x/y=w402:dbl[])
        n189 = Divide(x=w398, y=w391) -> (x/y=w403:dbl[])
        n190 = Natural Logarithm(1:w405) -> (0:w431:dbl[])
        n191 = Natural Logarithm(1:w401) -> (0:w430:dbl[])
        n192 = Natural Logarithm(1:w402) -> (0:w429:dbl[])
        n193 = Natural Logarithm(1:w403) -> (0:w428:dbl[])
        n194 = Array Subset(array=w431) -> (w426:dbl[])  [unwired: 2 in]
        n195 = Array Subset(array=w430) -> (w425:dbl[])  [unwired: 2 in]
        n196 = Array Subset(array=w429) -> (w424:dbl[])  [unwired: 2 in]
        n197 = Array Subset(array=w428) -> (w423:dbl[])  [unwired: 2 in]
        n198 = Array Subset(array=w427) -> (w422:dbl[])  [unwired: 2 in]
        n199 = Bundle(w422, w426) -> (w434:cluster{dbl[], dbl[]})  [unwired: 1 in]
        n200 = Bundle(w422, w425) -> (w436:cluster{dbl[], dbl[]})  [unwired: 1 in]
        n201 = Bundle(w422, w424) -> (w435:cluster{dbl[], dbl[]})  [unwired: 1 in]
        n202 = Bundle(w422, w423) -> (w433:cluster{dbl[], dbl[]})  [unwired: 1 in]
        n203 = Build Array(w434, w436, w435, w433) -> (w415:cluster{dbl[], dbl[]}[])
        n204 = call-poly <userlib>:"Linear Fit.vi"("XY-data"=w415) -> ("Best Fits"=w414:cluster{"X-array":dbl[], "Y-array":dbl[]}[], "XY-data out"=w413:cluster{"X-array":dbl[], "Y-array":dbl[]}[], "slopes"=w412:dbl[])  [unwired: 4 in, 4 out]
        n205 = Multiply(x=w412, y=8.617333e-05) -> (x*y=→"E_a":dbl[])
        n206 = Interleave 1D Arrays(w413, w414) -> (→"Arrhenius":cluster{"X-array":dbl[], "Y-array":dbl[]}[])
        n207 = call <vilib>:"Add State(s) to Queue__jki_lib_state_machine.vi"("State(s) in (\"\")"=w446) -> ("States Out"=w445:string)  [unwired: 14 in]
      }
    }
  }
  "error out" <- w3
  "Increasing Temp?" <- TRUE
  "Environment" <- enum16{"Air/Helium", "Vacuum"}."Vacuum" ("Environment")
